vi "Add_Inverse_Patterns_.vi"(1 "Hadamard":bool[][](array[boolean])) -> (0 "Array":bool[][](array[boolean]))   [LabVIEW 2020]
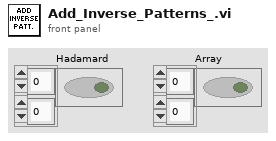
[diagram p1: front panel]
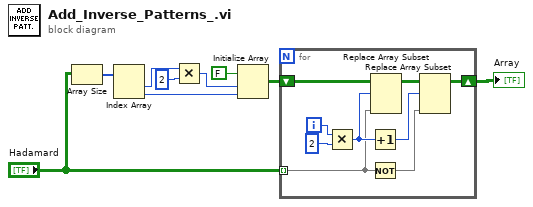
[diagram p0: block diagram]
diagram:
  n1 = Array Size(array="Hadamard") -> (size(s)=w5:i32[])
  n2 = Index Array(array=w5) -> (element #1=w7:i32, element #2=w9:i32)  [unwired: 2 in]
  n3 = Multiply(x=w7, y=2) -> (x*y=w8:i32)
  n4 = Initialize Array(FALSE, w8, w9) -> (w6:bool[][])
  n5 = for {
    tunnel: "Hadamard" -> [w11] mode=indexing
    shift-right: [w10] -> w1
    shift-left: w6 -> [w14]
    i -> [w17]
    n6 = Multiply(x=w17, y=2) -> (x*y=w16:i32)
    n7 = Increment(x=w16) -> (x+1=w15:i32)
    n8 = Not(x=w11) -> (.not. x?=w12:bool[])
    n9 = Replace Array Subset(array=w14, new element=w11, index (row)=w16) -> (w13:bool[][])  [unwired: 1 in]
    n10 = Replace Array Subset(array=w13, new element=w12, index (row)=w15) -> (w10:bool[][])  [unwired: 1 in]
  }
  "Array" <- w1
